vi "HoloPy_get_mean_std_var_volume.vi"(8 "error in (no error)":errorcluster, 11 "Refnum in":refnum<k35>) -> (0 "error out":errorcluster, 2 "data volume":cluster{"mean":dbl, "std var":dbl}, 3 "Refnum out":refnum<k35>)   [LabVIEW 2023, in "holoPyTracks.lvlib"]
uses:
  holoPyTracks.lvlib
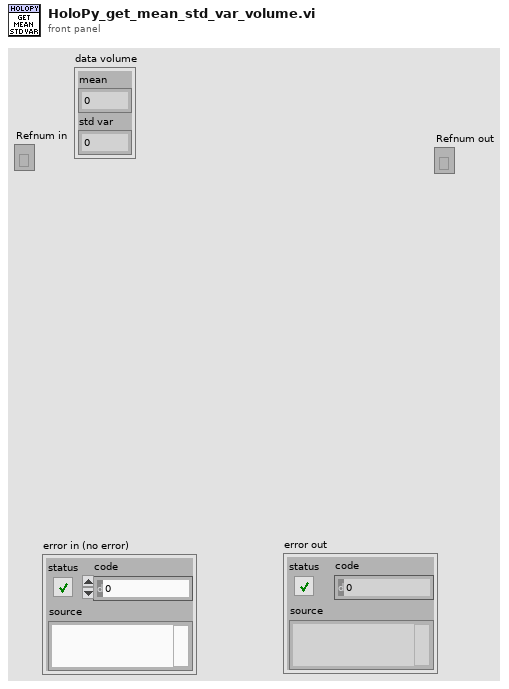
[diagram p1: front panel]
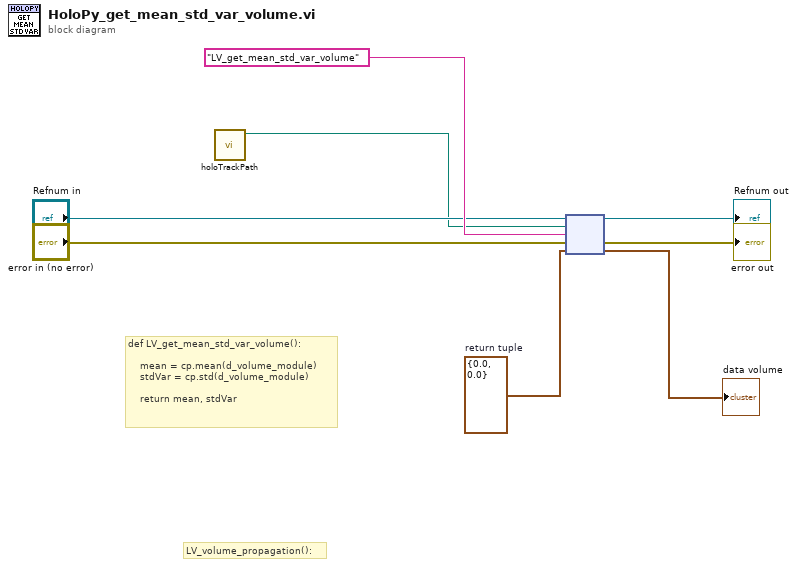
[diagram p0: block diagram]
diagram:
  w3 = cluster{"mean":dbl, "std var":dbl} {"mean"=0.0, "std var"=0.0}  # return tuple
  # "def LV_get_mean_std_var_volume():\n\n    mean = cp.mean(d_volume_module)\n    stdVar = cp.std(d_volume_module)\n\n    return mean, stdVar"
  # "LV_volume_propagation():"
  n1 = call "holoTrackPath.vi"() -> ("appended path"=w1:path)  [unwired: 11 in]
  n2 = node("Refnum in", w1, "LV_get_mean_std_var_volume" ("function name"), "error in (no error)", w3) -> (→"Refnum out":refnum<k35>, →"error out":errorcluster, →"data volume":cluster{"mean":dbl, "std var":dbl})  [unwired: 2 out]
